vi "Connect Manager.vi"(6 "Server Certificate File (.crt)":path, 8 "error in (no error)":errorcluster, 9 "VI Reference":refnum<vi>, 10 "Address":string, 11 "CIF_UI in":refnum<class "CIF_UI.lvclass">) -> (0 "error out":errorcluster, 3 "CIF_UI out":refnum<class "CIF_UI.lvclass">)   [LabVIEW 2021, in "CIF_UI.lvclass"]
uses:
  CIF_UI.lvclass
  Typedef/Plugin Connection Map.ctl
  Typedef/Plugin Connections.ctl
  <vilib>/gRPC/LabVIEW gRPC Library/Shared/grpcId.ctl
  Typedef/PluginInfo.ctl
  Typedef/Version.ctl
  CIFCore/Common/Typedef/gRPC Reported Plugin Status.ctl
  CIFCore/Common/Typedef/Plugin State.ctl
  CIFCore/Common/Typedef/Timing Statistics.ctl
  CIFCore/Common/Typedef/Timing Stats Base.ctl
  CIFCore/Common/Typedef/FIFO Statistics.ctl
  CIFCore/Common/Typedef/Simple Error.ctl
  CIFCore/Common/Typedef/Monitor Doubles.ctl
  CIFCore/Common/Typedef/Monitor U64.ctl
  CIFCore/Common/Typedef/Monitor I64.ctl
  CIFCore/Common/Typedef/Errors.ctl
  CIF_UI.lvclass/CIF_UI.ctl
  <vilib>/CIF Foundation/CIF Utilities/Errors/Append Error Location.vi
  CIFPluginManager/CIFPluginManager/gRPC/CIF_Manager_Client_Wrapper/CIFManagerClientWrapper.lvlib
  <vilib>/gRPC/LabVIEW gRPC Library/grpc-lvsupport-release.lvlib
  CIFCore/Common/CIFCoreCommon.lvlib
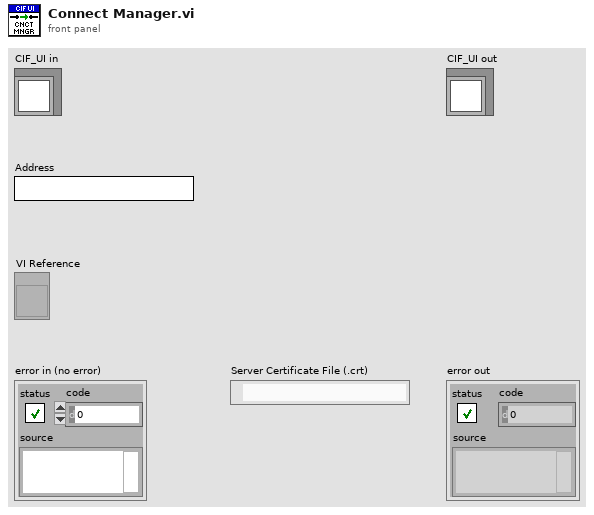
[diagram p1: front panel]
types:
  T1 = typedef "CIFCoreCommon.lvlib/Errors.ctl" = enum16{"Invalid Clock ID", "Long Sleep", "gRPC Server Not Found", "Config Parse", "Timestamp Wrap", "Delayed Execution", "Duplicate Channel", "Missing Channel", "Incorrect Type", "Flatten Error", "Unflatten Data", "Unique Name", "Plugin Not Found", "Plugin Type Not Found", "Plugin Version Not Found", "Manager Not Found", "Numerical Issue", "Time Jump", "Clock ID Match", "Channel Length", "Plugin Connection", "gRPC Server Connection", "PPL Name Match", "Build", "Config Log Parse", "Plugin Load"}
  T2 = typedef "CIF_UI.lvclass/Plugin Connection Map.ctl" = map{string, T3}
  T3 = typedef "CIF_UI.lvclass/Plugin Connections.ctl" = cluster{"gRPC ID":T4, "Plugin Info":T5}
  T4 = typedef "grpc-lvsupport-release.lvlib/grpcId.ctl" = u64
  T5 = typedef "CIF_UI.lvclass/PluginInfo.ctl" = cluster{"Name":string, "Type":string, "grpc_port":i32, "Version":T6, "Node Status":T7}
  T6 = typedef "CIF_UI.lvclass/Version.ctl" = cluster{"Major":i32, "Minor":i32, "Fix":i32}
  T7 = typedef "CIFCoreCommon.lvlib/gRPC Reported Plugin Status.ctl" = cluster{"State":T8, "Timing Statistics (us)":T9, "FIFO Statistics (us)":T11, "error":T12, "Monitor Doubles":T13, "Monitor U64":T14, "Monitor I64":T15}
  T8 = typedef "CIFCoreCommon.lvlib/Plugin State.ctl" = enum32{"Null", "Creating", "Listening", "Running", "CleaningUp", "Destroying"}
  T9 = typedef "CIFCoreCommon.lvlib/Timing Statistics.ctl" = cluster{"Period":T10, "Wake Error":T10, "Execute":T10, "Housekeep":T10, "Idle":T10, "Cleanup":T10, "Custom 1 (custom units)":T10, "Custom 2 (custom units)":T10}
  T10 = typedef "CIFCoreCommon.lvlib/Timing Stats Base.ctl" = cluster{"Max":i64, "Avg":dbl, "Min":i64}
  T11 = typedef "CIFCoreCommon.lvlib/FIFO Statistics.ctl" = cluster{"From T0":T10, "From Previous Plugin":T10, "Output Error":T10}
  T12 = typedef "CIFCoreCommon.lvlib/Simple Error.ctl" = cluster{"status":bool, "code":i32}
  T13 = typedef "CIFCoreCommon.lvlib/Monitor Doubles.ctl" = cluster{"1":dbl, "2":dbl, "3":dbl, "4":dbl}
  T14 = typedef "CIFCoreCommon.lvlib/Monitor U64.ctl" = cluster{"1":u64, "2":u64, "3":u64, "4":u64}
  T15 = typedef "CIFCoreCommon.lvlib/Monitor I64.ctl" = cluster{"1":i64, "2":i64, "3":i64, "4":i64}
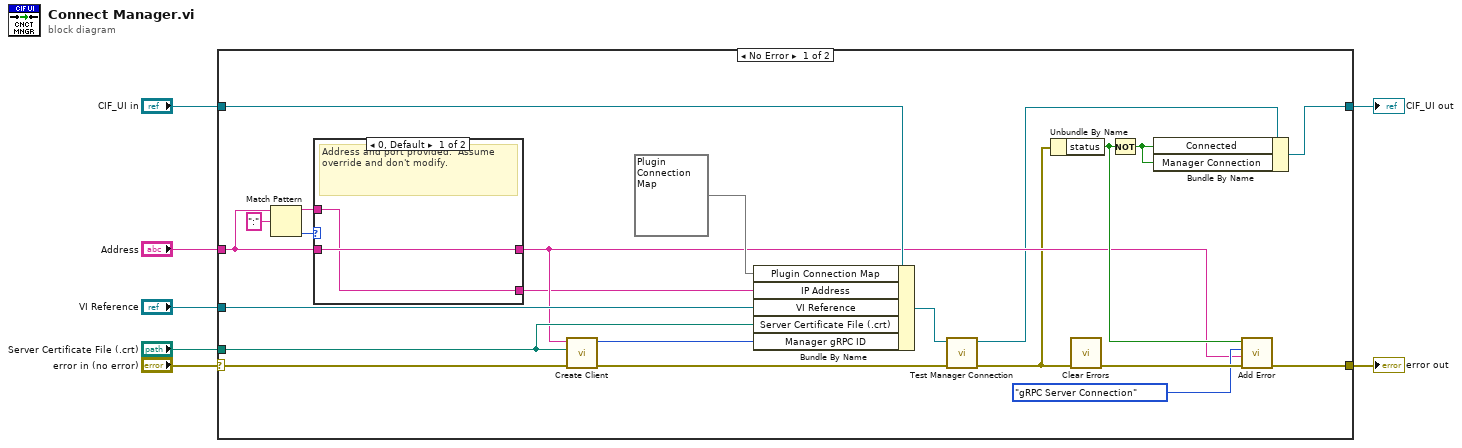
[diagram p0: block diagram]
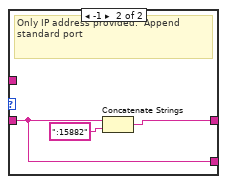
[diagram p2: hidden frame]
diagram:
  n1 = case shown="No Error" "error in (no error)" {
    selector: "error in (no error)" -> [w27 w36]
    tunnel: [w8 w36] -> w6
    tunnel: [w9 w35] -> w4
    tunnel: "CIF_UI in" -> [w28 w35]
    tunnel: "Address" -> [w24 _]
    tunnel: "VI Reference" -> [w29 _]
    tunnel: "Server Certificate File (.crt)" -> [w23 _]
    frame No Error {
      n2 = Match Pattern(string=w24, regular expression=":") -> (before substring=w11:string, offset past match=w26:i32)  [unwired: 1 in, 2 out]
      n3 = case shown="0, Default" w26 {
        tunnel: w24 -> [w31 w32]
        tunnel: [w31 w34] -> w17
        tunnel: [w30 w32] -> w12
        tunnel: w11 -> [w30 _]
        frame 0, Default {
          # "Address and port provided.  Assume override and don't modify."
        }
        frame -1 {
          # "Only IP address provided.  Append standard port"
          n4 = Concatenate Strings(w32, ":15882" ("string")) -> (w34:string)
        }
      }
      n5 = call "Create Client.vi"("error in"=w27, "Server Certificate File (.crt)"=w23, "address"=w17) -> ("error out"=w15:errorcluster, "gRPC ID Out"=w21:T4)  [unwired: 7 in]
      n6 = Bundle By Name(cluster=w28, "Plugin Connection Map"=T2 {}, "IP Address"=w12, "VI Reference"=w29, "Server Certificate File (.crt)"=w23, "Manager gRPC ID"=w21) -> (w16:refnum<class "CIF_UI.lvclass">)
      n7 = call "Test Manager Connection.vi"("error in (no error)"=w15, "CIF_UI in"=w16) -> ("error out"=w14:errorcluster, "CIF_UI out"=w13:refnum<class "CIF_UI.lvclass">)  [unwired: 8 in]
      n8 = Unbundle By Name(w14) -> ("status"=w19:bool)
      n9 = call <vilib>:"Clear Errors.vi"("error in (no error)"=w14) -> ("error out"=w20:errorcluster)  [unwired: 5 in, 1 out]
      n10 = Not(x=w19) -> (.not. x?=w10:bool)
      n11 = Bundle By Name(cluster=w13, "Connected"=w10, "Manager Connection"=w10) -> (w9:refnum<class "CIF_UI.lvclass">)
      n12 = call "Add Error.vi"("error in (no error)"=w20, "String to Append"=w17, "Error"=Errors."gRPC Server Connection", "Insert Error"=w19) -> ("error out"=w8:errorcluster)  [unwired: 7 in]
    }
    frame Error {
    }
  }
  "error out" <- w6
  "CIF_UI out" <- w4
